vi "Read Old Mentions - Finite.vi"() -> ()   [LabVIEW 2011]
doc: "This example gets a finite number of mentions starting from the top of of the user's timeline."
uses:
  Controls/Tweet.ctl
  SubVIs/Twitter Open - Desktop.vi
  Mentions/Get Mentions Old.vi
  i3-twitter.lvlib
panel:
  out "Mentions":T1[](array[typedef])
  out "Time Stamp of Oldest Mention":timestamp
  out "Num of Mentions Read":i32
  in  "Num of Mentions to Read":i32=10
  in  "Consumer Key":string
  in  "Consumer Secret":string
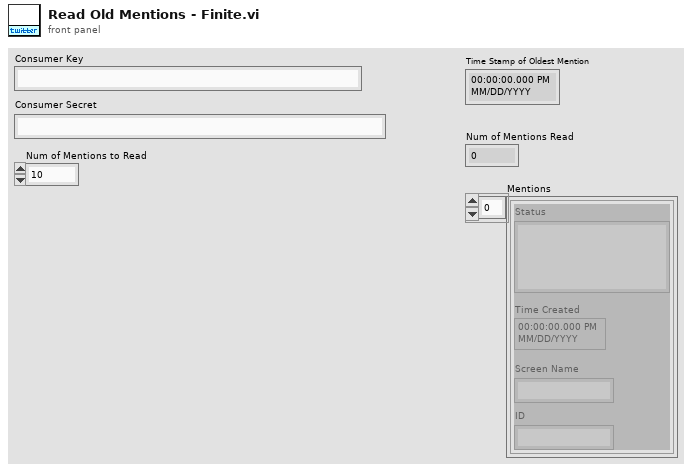
[diagram p1: front panel]
types:
  T1 = typedef "i3-twitter.lvlib/Tweet.ctl" = cluster{"Status":string, "Time Created":timestamp, "Screen Name":string, "ID":string}
  T2 = typedef "i3-oauth.lvlib/Credentials.ctl" = cluster{"Token":string, "Secret":string}
  T3 = typedef "i3-twitter.lvlib/Twitter Handle.ctl" = cluster{"OAuth Credentials":T4, "since ID":string, "max ID":string, "Screen Name":string}
  T4 = typedef "i3-oauth.lvlib/OAuth Handle.ctl" = cluster{"Signature Method":T5, "Version":string, "Client":T2, "Access":T2}
  T5 = typedef "i3-oauth.lvlib/Signature Method.ctl" = enum16{"HMAC-MD5", "HMAC-SHA1", "HMAC-SHA224", "HMAC-SHA256", "HMAC-SHA384", "HMAC-SHA512"}
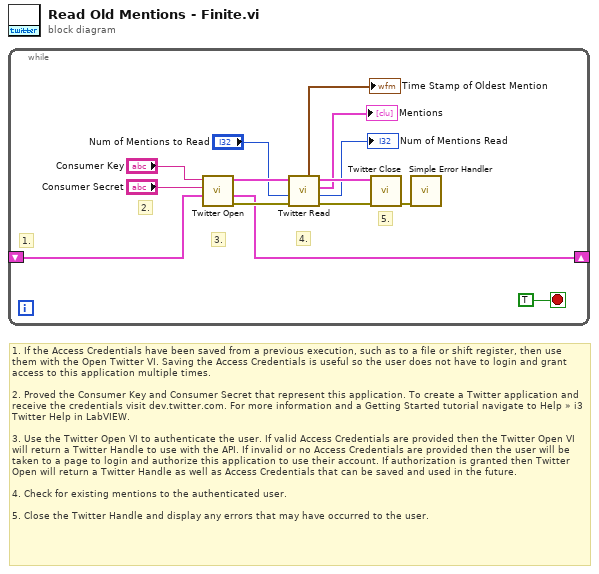
[diagram p0: block diagram]
diagram:
  # "1. If the Access Credentials have been saved from a previous execution, such as to a file or shift register, then use them with the Open Twitter VI. Saving the Access Credentials is useful so the user does not have to login and grant access to this application multiple times.\n\n2. Proved the Consumer Key and Consumer Secret that represent this application. To create a Twitter application and receive the credentials visit dev.twitter.com. For more information and a Getting Started tutorial navigate to Help » i3 Twitter Help in LabVIEW.\n\n3. Use the Twitter Open VI to authenticate the user. If valid Access Credentials are provided then the Twitter Open VI will return a Twitter Handle to use with the API. If invalid or no Access Credentials are provided then the user will be taken to a page to login and authorize this application to use their account. If authorization is granted then Twitter Open will return a Twitter Handle as well as Access Credentials that can be saved and used in the future.\n\n4. Check for existing mentions to the authenticated user.\n\n5. Close the Twitter Handle and display any errors that may have occurred to the user."
  n1 = while {
    shift-right: [w2] -> _
    shift-left: _ -> [w1]
    stop <- TRUE stop-if-true
    # "5."
    # "4."
    # "3."
    # "2."
    # "1."
    n2 = call-poly "Twitter Open.vi"("Access Credentials (in)"=w1, "Consumer Secret"="Consumer Secret", "Consumer Key"="Consumer Key") -> ("error out"=w9:errorcluster, "Access Credentials (out)"=w2:T2, "Twitter Handle Out"=w12:T3)  [unwired: 6 in]
    n3 = call-poly "Twitter Read.vi"("error in"=w9, "Mentions to Read (10)"="Num of Mentions to Read", "Twitter Handle In"=w12) -> ("error out"=w11:errorcluster, "Actual Num of Mentions Read"=→"Num of Mentions Read":i32, "Old Mentions Read"=→"Mentions":T1[], "Twitter Handle Out"=w10:T3, "Time Stamp of Oldest Mention"=→"Time Stamp of Oldest Mention":timestamp)  [unwired: 4 in]
    n4 = call "Twitter Close.vi"("error in"=w11, "Twitter Handle In"=w10) -> ("error out"=w5:errorcluster)  [unwired: 9 in]
    n5 = call <vilib>:"Simple Error Handler.vi"("error in (no error)"=w5) -> ()  [unwired: 4 in, 5 out]
  }
